vi "Lock-in.vi"() -> ()   [LabVIEW 2014]
uses:
  <vilib>/express/express shared/transition.llb/Dynamic To Waveform Array.vi
  <vilib>/express/express arith-compare/Formula/Block/exnFormulaBlock how many pts in the wave.vi
  <vilib>/express/express shared/ex_Modify Signal Name.vi
  <vilib>/express/express shared/transition.llb/Waveform Array To Dynamic.vi
  <vilib>/Utility/file.llb/Write To Spreadsheet File (DBL).vi
  <vilib>/express/express arith-compare/Formula/XNode/ExpressFormulaBlockNode.xnode
panel:
  in  "Write":bool
  out "Handled Signal":dynamicdata(graph)
  out "Input Signal":dynamicdata(graph)
  in  "?":bool
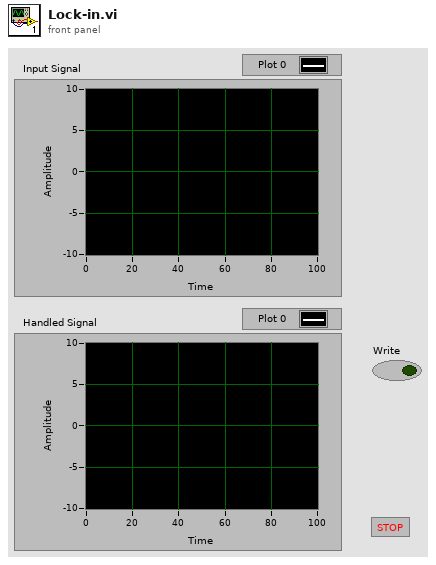
[diagram p1: front panel]
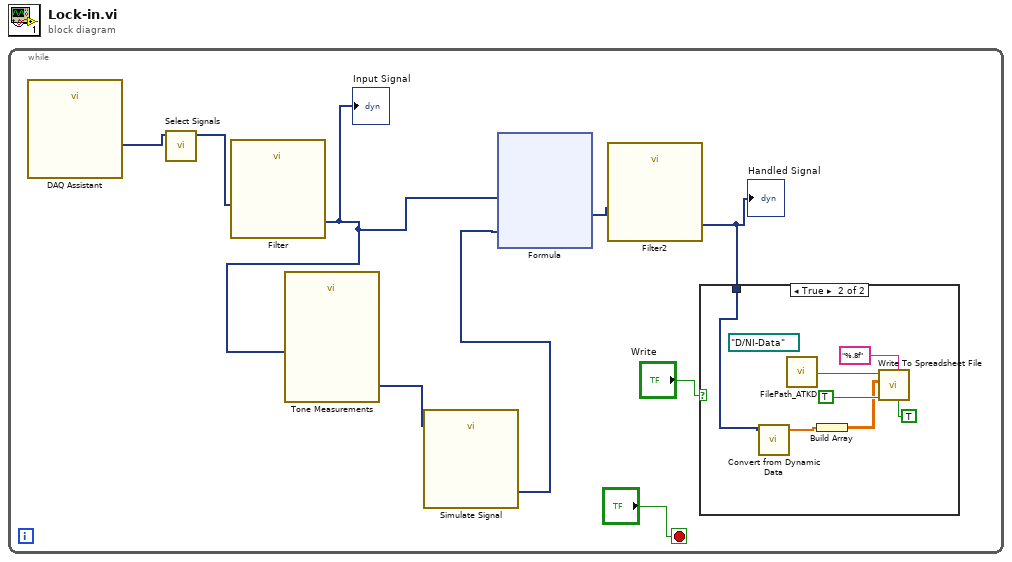
[diagram p0: block diagram]
diagram:
  n1 = while {
    stop <- "?" stop-if-true
    n2 = call "DAQ Assistant"() -> ("data"=w9:dynamicdata)  [unwired: 2 in, 9 out]
    n3 = call "Select Signals"("Signals"=w9) -> ("Signal Out"=w8:dynamicdata)  [unwired: 1 in, 9 out]
    n4 = call "Filter"("Signal"=w8) -> ("Filtered Signal"=w4:dynamicdata)  [unwired: 9 in, 1 out]
    "Input Signal" <- w4
    n5 = call "Tone Measurements"("Signals"=w4) -> ("Frequency"=w7:dynamicdata)  [unwired: 8 in, 2 out]
    n6 = call "Simulate Signal"("Frequency"=w7) -> ("Sine"=w6:dynamicdata)  [unwired: 13 in, 1 out]
    n7 = xnode "Formula"("Signal"=w4, "Sine"=w6) -> ("Result"=w3:dynamicdata)  [unwired: 1 in, 1 out]
    n8 = call "Filter2"("Signal"=w3) -> ("Filtered Signal"=w1:dynamicdata)  [unwired: 9 in, 1 out]
    "Handled Signal" <- w1
    n9 = case shown="True" "Write" {
      tunnel: w1 -> [_ w11]
      frame False {
      }
      frame True {
        (unwired) path "D:/NI-Data" ("base folder path")
        n10 = call "Convert from Dynamic Data"("Dynamic Data Type"=w11) -> ("Array"=w12:dbl[])  [unwired: 3 out]
        n11 = call "FilePath_ATKD.vi"() -> ("ATKD"=w13:path)  [unwired: 1 in, 3 out]
        n12 = Build Array(w12) -> (w10:dbl[][])
        n13 = call-poly <vilib>:"Write To Spreadsheet File.vi"("transpose? (no:F)"=TRUE, "format (%.3f)"="%.8f", "append to file? (new file:F)"=TRUE, "2D data"=w10, "file path (dialog if empty)"=w13) -> ()  [unwired: 1 in, 3 out]
      }
    }
  }
